vi "Map Store.vi"(7 "Cursor List":T4, 8 "error in (no error)":errorcluster, 9 "Data File":path, 10 "All Lines":T1, 11 "Command":T5) -> (0 "error out":errorcluster, 1 "Cursor List":T4, 2 "Data Modified?":bool, 3 "All Lines out":T1)   [LabVIEW 2014, in "Map Data.lvlib"]
doc: "The main action engine VI that stores the address book data using functional global variables."
uses:
  Map Data.lvlib
  MapCommand.ctl
  CursorList.ctl
  All-Lines.ctl
  LineCluster.ctl
  LineConnection.ctl
  MapData.ctl
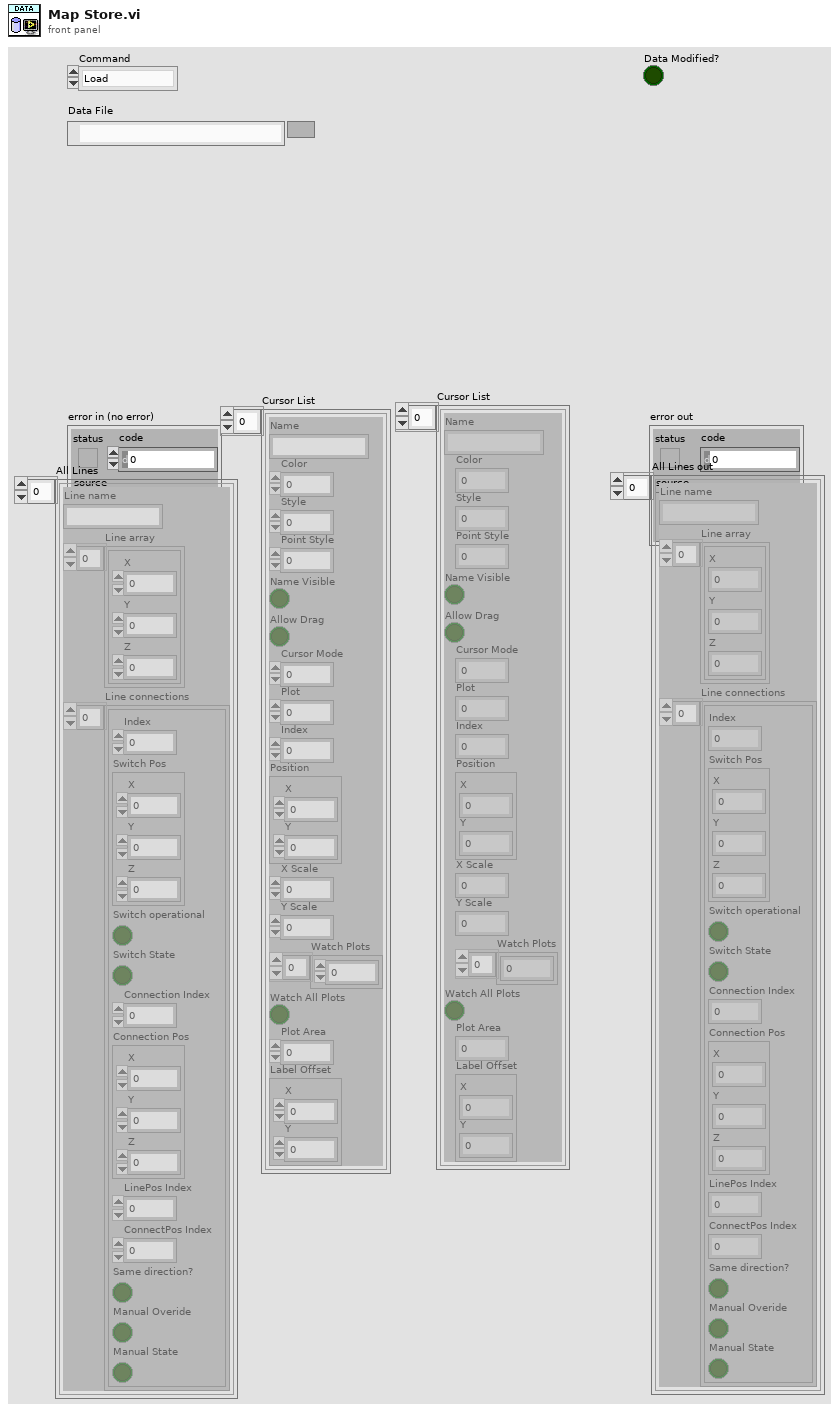
[diagram p1: front panel]
types:
  T1 = typedef "Map Data.lvlib/All-Lines.ctl" = T2[]
  T2 = typedef "Map Data.lvlib/LineCluster.ctl" = cluster{"Line name":string, "Line array":cluster{"X":dbl, "Y":dbl, "Z":dbl}[], "Line connections":T3[]}
  T3 = typedef "Map Data.lvlib/LineConnection.ctl" = cluster{"Index":i32, "Switch Pos":cluster{"X":dbl, "Y":dbl, "Z":dbl}, "Switch operational":bool, "Switch State":bool, "Connection Index":i32, "Connection Pos":cluster{"X":dbl, "Y":dbl, "Z":dbl}, "LinePos Index":i32, "ConnectPos Index":i32, "Same direction?":bool, "Manual Overide":bool, "Manual State":bool}
  T4 = typedef "Map Data.lvlib/CursorList.ctl" = cluster{"Name":string, "Color":u32, "Style":u8, "Point Style":u8, "Name Visible":bool, "Allow Drag":bool, "Cursor Mode":u32, "Plot":i32, "Index":i32, "Position":cluster{"X":dbl, "Y":dbl}, "X Scale":u32, "Y Scale":u32, "Watch Plots":i32[], "Watch All Plots":bool, "Plot Area":i32, "Label Offset":cluster{"X":dbl, "Y":dbl}}[]
  T5 = typedef "Map Data.lvlib/MapCommand.ctl" = enum16{"Load", "Update Cursor", "Save", "Get All Data", "Get Single Data", "Set Single Data", "Delete All", "Remove Single Data", "Set Favorite Status", "Is Data Modified", "Import Data"}
  T6 = typedef "Map Data.lvlib/MapData.ctl" = cluster{"Last ID":u32, "Cursor List":T4, "All Lines":T1}
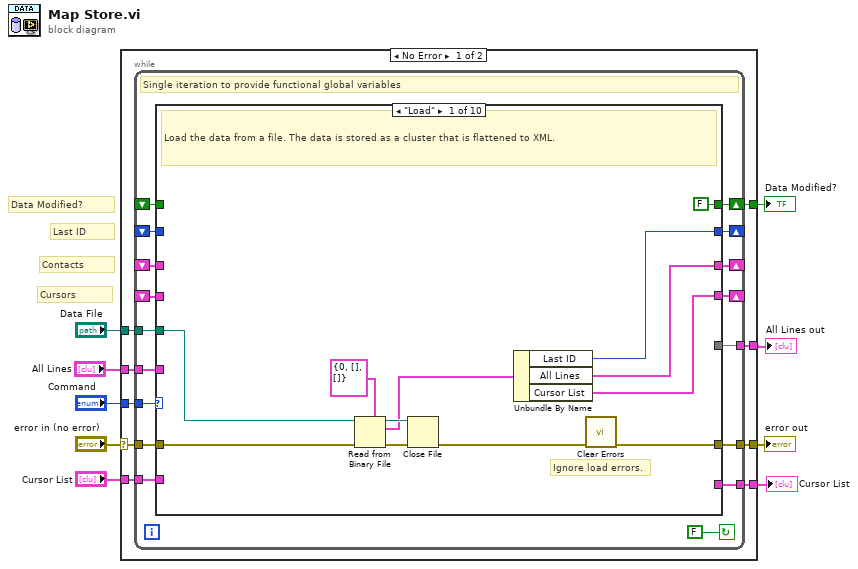
[diagram p0: block diagram]
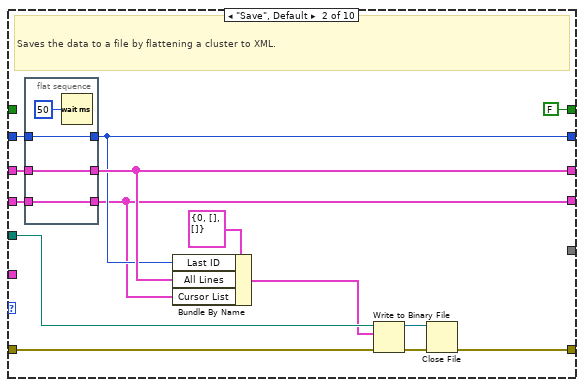
[diagram p2: hidden frame]
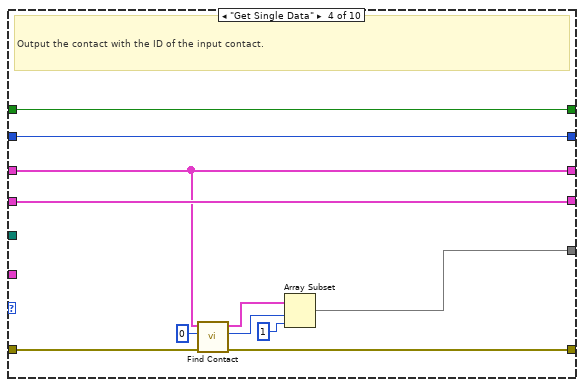
[diagram p4: hidden frame]
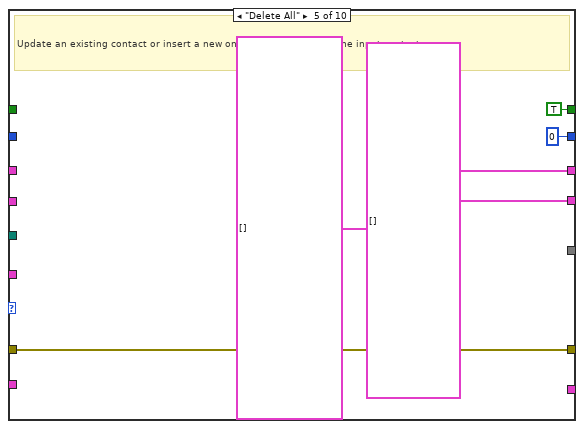
[diagram p5: hidden frame]
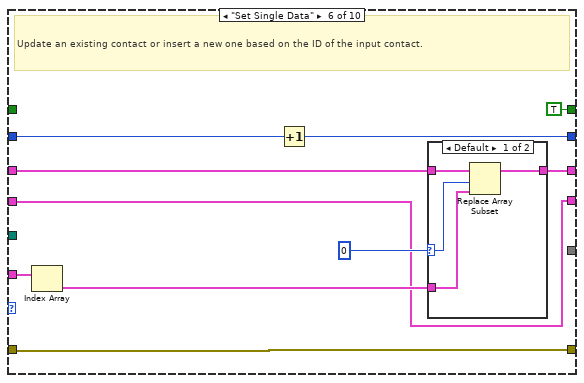
[diagram p6: hidden frame]
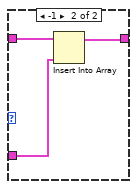
[diagram p7: hidden frame]
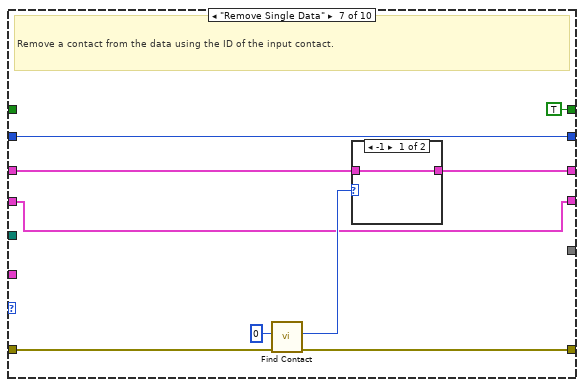
[diagram p8: hidden frame]
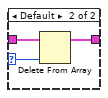
[diagram p9: hidden frame]
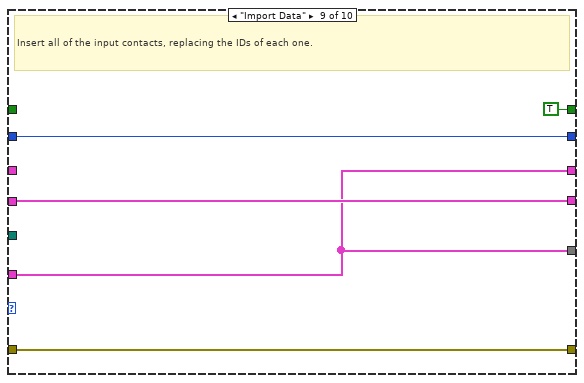
[diagram p11: hidden frame]
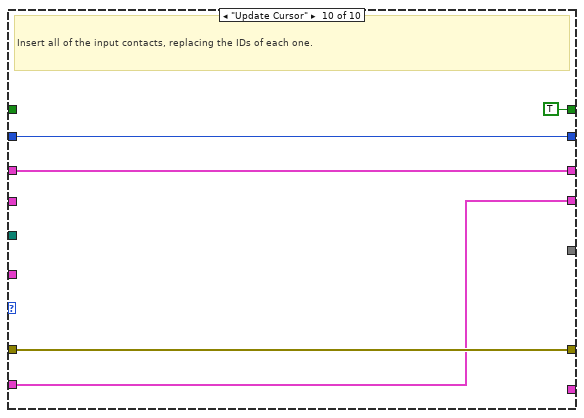
[diagram p12: hidden frame]
diagram:
  # "Cursors"
  # "Contacts"
  # "Last ID"
  # "Data Modified?"
  n1 = case shown="No Error" "error in (no error)" {
    selector: "error in (no error)" -> [w17 w133]
    tunnel: [w18 w133] -> w9
    tunnel: "Command" -> [w16 _]
    tunnel: "All Lines" -> [w15 w132]
    tunnel: [w14 w132] -> w2
    tunnel: "Data File" -> [w13 _]
    tunnel: [w12 _] -> w5
    tunnel: "Cursor List" -> [w11 _]
    tunnel: [w10 _] -> w3
    frame No Error {
      n2 = while {
        tunnel: [w34] -> w18
        tunnel: w17 -> [w33]
        tunnel: w16 -> [w30]
        tunnel: w15 -> [w23]
        shift-right: [w35] -> _
        shift-left: _ -> [w28]
        shift-right: [w31] -> _
        shift-left: _ -> [w32]
        tunnel: [w27] -> w14
        shift-right: [w26] -> w12
        shift-left: _ -> [w25]
        tunnel: w13 -> [w24]
        shift-right: [w22] -> _
        shift-left: _ -> [w21]
        tunnel: w11 -> [w20]
        tunnel: [w19] -> w10
        stop <- FALSE continue-if-true
        # "Single iteration to provide functional global variables"
        n3 = case shown="\"Load\"" w30 {
          tunnel: w33 -> [w46 w53 w69 w81 w85 w91 w108 w118 w126 w131]
          tunnel: [w43 w49 w69 w78 w85 w91 w107 w118 w126 w131] -> w34
          tunnel: w28 -> [_ w59 w68 w72 _ w95 w104 w121 _ w128]
          tunnel: [w41 w58 w68 w72 T1 [] ("All Lines") w94 w111 w121 w122 w128] -> w35
          tunnel: w23 -> [_ _ _ _ _ w90 _ _ w122 _]
          tunnel: w32 -> [_ w56 w70 w79 _ w89 w110 w120 w125 w130]
          tunnel: [w45 w57 w70 w79 u32 0 ("Last ID") w93 w110 w120 w125 w130] -> w31
          tunnel: [FALSE FALSE w67 w77 TRUE TRUE TRUE w119 TRUE TRUE] -> w26
          tunnel: [_ _ w68 w71 _ _ _ _ w122 _] -> w27
          tunnel: w25 -> [_ _ w67 w77 _ _ _ w119 _ _]
          tunnel: w24 -> [w44 w52 _ _ _ _ _ _ _ _]
          tunnel: [w42 w54 w66 w74 T4 [] ("Cursor List") w87 w105 w117 w124 w129] -> w22
          tunnel: w21 -> [_ w55 w66 w74 _ w87 w105 w117 w124 _]
          tunnel: w20 -> [_ _ _ _ _ _ _ _ _ w129]
          tunnel: [_ _ w66 _ _ _ _ _ _ _] -> w19
          frame "Load" {
            # "Ignore load errors."
            # "Load the data from a file. The data is stored as a cluster that is flattened to XML."
            n4 = Read from Binary File(5:T6 {"Last ID"=0, "Cursor List"=[], "All Lines"=[]} ("Data"), 8:w46, 11:w44) -> (0:w39:errorcluster, 2:w36:T6, 3:w38:refnum<file>)  [unwired: 3 in, 1 out]
            n5 = Close File(refnum=w38, error in=w39) -> (error out=w37:errorcluster)  [unwired: 1 out]
            n6 = Unbundle By Name(w36) -> ("Last ID"=w45:u32, "All Lines"=w41:T1, "Cursor List"=w42:T4)
            n7 = call <vilib>:"Clear Errors.vi"("error in (no error)"=w37) -> ("error out"=w43:errorcluster)  [unwired: 5 in, 1 out]
          }
          frame "Save", Default {
            # "Saves the data to a file by flattening a cluster to XML."
            n8 = flat-sequence {
              tunnel: w59 -> [w64]
              tunnel: [w64] -> w58
              tunnel: [w63] -> w57
              tunnel: w56 -> [w63]
              tunnel: w55 -> [w62]
              tunnel: [w62] -> w54
              frame #0 {
                n9 = Wait (ms)(milliseconds to wait=u32 50) -> ()  [unwired: 1 out]
              }
            }
            n10 = Bundle By Name(cluster=T6 {"Last ID"=0, "Cursor List"=[], "All Lines"=[]} ("File Data"), "Last ID"=w57, "All Lines"=w58, "Cursor List"=w54) -> (w48:T6)
            n11 = Write to Binary File(file (use dialog)=w52, data=w48, error in=w53) -> (refnum out=w51:refnum<file>, error out=w50:errorcluster)  [unwired: 3 in, 1 out]
            n12 = Close File(refnum=w51, error in=w50) -> (error out=w49:errorcluster)  [unwired: 1 out]
          }
          frame "Get All Data" {
            # "Output all of the contact data."
          }
          frame "Get Single Data" {
            # "Output the contact with the ID of the input contact."
            n13 = call "Find Contact.vi"("error in (no error)"=w81, "ID"=u32 0, "All Lines"=w72) -> ("error out"=w78:errorcluster, "Index"=w80:i32, "All Lines 2"=w73:T1)  [unwired: 6 in]
            n14 = Array Subset(array=w73, index=w80, length=1) -> (w71:T1)
          }
          frame "Delete All" {
            # "Update an existing contact or insert a new one based on the ID of the input contact."
          }
          frame "Set Single Data" {
            # "Update an existing contact or insert a new one based on the ID of the input contact."
            n15 = Index Array(array=w90) -> (element=w88:T2)  [unwired: 1 in]
            n16 = Increment(x=w89) -> (x+1=w93:u32)
            n17 = case shown="Default" 0 ("Index") {
              selector: 0 ("Index") -> [w98 _]
              tunnel: w95 -> [w100 w103]
              tunnel: w88 -> [w99 w101]
              tunnel: [w97 w102] -> w94
              frame Default {
                n18 = Replace Array Subset "Replace Array Subset"(array=w100, new element=w99, index=w98) -> (w97:T1)
              }
              frame -1 {
                n19 = Insert Into Array(array=w103, new element=w101) -> (w102:T1)  [unwired: 1 in]
              }
            }
          }
          frame "Remove Single Data" {
            # "Remove a contact from the data using the ID of the input contact."
            n20 = call "Find Contact.vi"("error in (no error)"=w108, "ID"=u32 0) -> ("error out"=w107:errorcluster, "Index"=w112:i32)  [unwired: 7 in, 1 out]
            n21 = case shown="-1" w112 {
              selector: w112 -> [_ w115]
              tunnel: w104 -> [w113 w116]
              tunnel: [w113 w114] -> w111
              frame -1 {
              }
              frame Default {
                n22 = Delete From Array(array=w116, index=w115) -> (array with subset deleted=w114:T1)  [unwired: 1 in, 1 out]
              }
            }
          }
          frame "Is Data Modified" {
            # "Output if the data has been modified or not since the last save command."
          }
          frame "Import Data" {
            # "Insert all of the input contacts, replacing the IDs of each one."
          }
          frame "Update Cursor" {
            # "Insert all of the input contacts, replacing the IDs of each one."
          }
        }
      }
    }
    frame Error {
    }
  }
  "error out" <- w9
  "Data Modified?" <- w5
  "Cursor List" <- w3
  "All Lines out" <- w2
